vi "HEWH Standard ERD List.vi"(8 "Error In":errorcluster, 11 "Disable ERD (Main)":bool) -> (0 "Error Out":errorcluster, 2 "Header":string[](array[string]), 3 "Read ERD List":T1[](array[typedef]) {"ERD Number" format="%.0x"})   [LabVIEW 2016]
uses:
  type defs/ERD Read Data In.ctl
  type defs/Data Type.ctl
  library/GEA2_Toolkit.lvlib
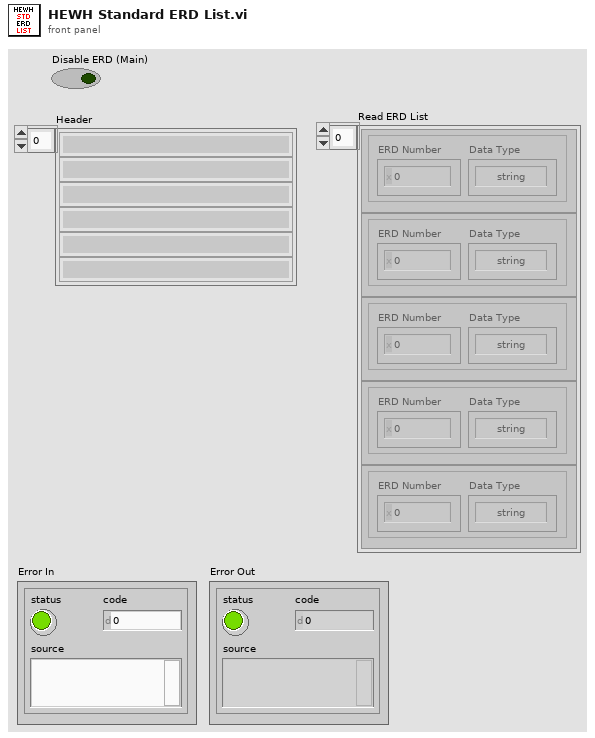
[diagram p1: front panel]
types:
  T1 = typedef "GEA2_Toolkit.lvlib/ERD Read Data In.ctl" = cluster{"ERD Number":u16, "Data Type":T2}
  T2 = typedef "GEA2_Toolkit.lvlib/Data Type.ctl" = enum16{"string", "boolean", "uint8_t", "uint16_t", "uint32_t", "uint64_t"}
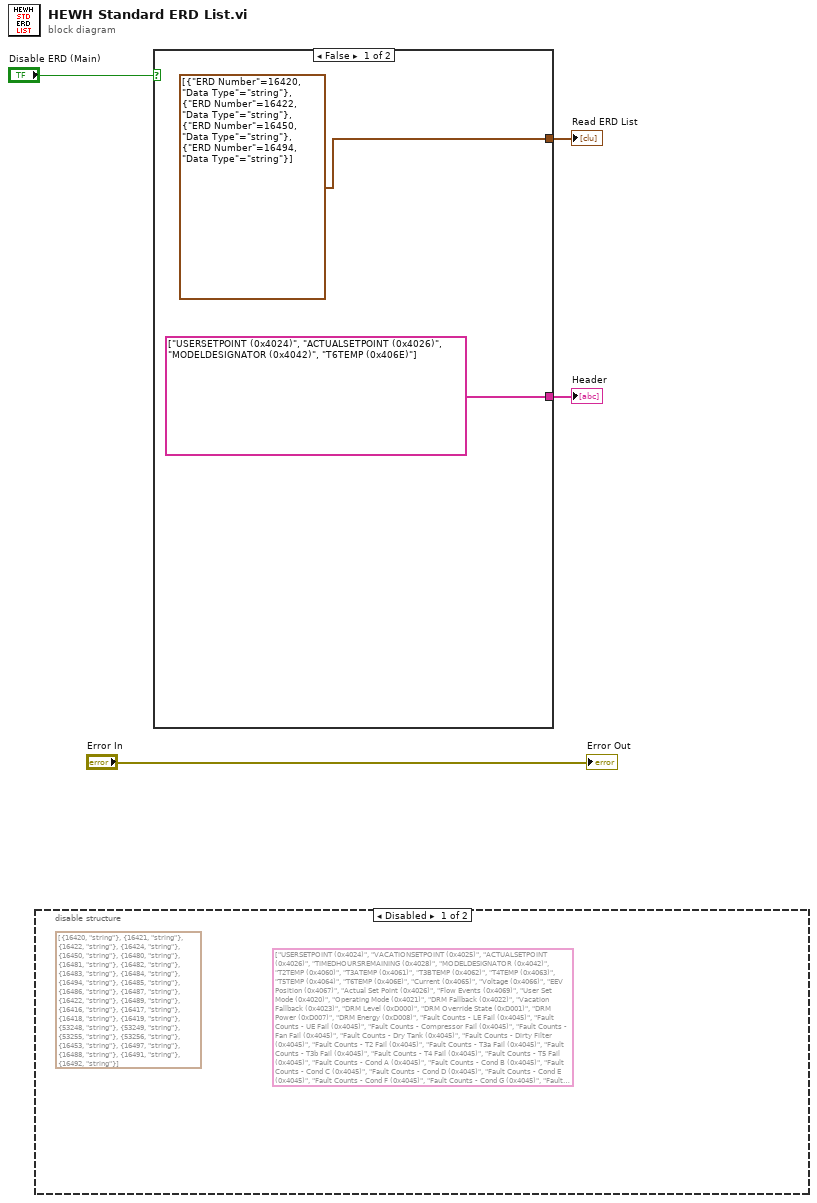
[diagram p0: block diagram]
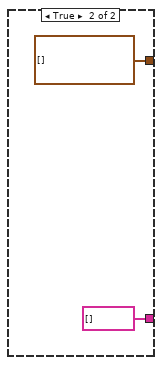
[diagram p3: hidden frame]
diagram:
  n1 = disable-structure shown="Disabled" {
    frame Disabled {
      (unwired) string[] ["USERSETPOINT (0x4024)", "VACATIONSETPOINT (0x4025)", "ACTUALSETPOINT (0x4026)", "TIMEDHOURSREMAINING (0x4028)", "MODELDESIGNATOR (0x4042)", "T2TEMP (0x4060)", "T3ATEMP (0x4061)", "T3BTEMP (0x4062)", "T4TEMP (0x4063)", "T5TEMP (0x4064)", "T6TEMP (0x406E)", "Current (0x4065)", "Voltage (0x4066)", "EEV Position (0x4067)", "Actual Set Point (0x4026)", "Flow Events (0x4069)", "User Set Mode (0x4020)", "Operating Mode (0x4021)", "DRM Fallback (0x4022)", "Vacation Fallback (0x4023)", "DRM Level (0xD000)", "DRM Override State (0xD001)", "DRM Power (0xD007)", "DRM Energy (0xD008)", "Fault Counts - LE Fail (0x4045)", "Fault Counts - UE Fail (0x4045)", "Fault Counts - Compressor Fail (0x4045)", "Fault Counts - Fan Fail (0x4045)", "Fault Counts - Dry Tank (0x4045)", "Fault Counts - Dirty Filter (0x4045)", "Fault Counts - T2 Fail (0x4045)", "Fault Counts - T3a Fail (0x4045)", "Fault Counts - T3b Fail (0x4045)", "Fault Counts - T4 Fail (0x4045)", "Fault Counts - T5 Fail (0x4045)", "Fault Counts - Cond A (0x4045)", "Fault Counts - Cond B (0x4045)", "Fault Counts - Cond C (0x4045)", "Fault Counts - Cond D (0x4045)", "Fault Counts - Cond E (0x4045)", "Fault Counts - Cond F (0x4045)", "Fault Counts - Cond G (0x4045)", "Fault Counts - Cond H (0x4045)", "Fault Counts - Cond I (0x4045)", "Fault Counts - Cond J (0x4045)", "Fault Counts - Cond L (0x4045)", "Condensate Drain Pan Voltage (0x4071)", "Relay States - DLB (0x4068)", "Relay States - Compressor (0x4068)", "Relay States - Upper Element (0x4068)", "Relay States - Lower Element (0x4068)", "Relay States - Fan (0x4068)", "Compressor Min On/Off Time (0x406B)", "SS Run State (0x406C)"]
      (unwired) T1[] [{"ERD Number"=16420, "Data Type"=enum."string"}, {"ERD Number"=16421, "Data Type"=enum."string"}, {"ERD Number"=16422, "Data Type"=enum."string"}, {"ERD Number"=16424, "Data Type"=enum."string"}, {"ERD Number"=16450, "Data Type"=enum."string"}, {"ERD Number"=16480, "Data Type"=enum."string"}, {"ERD Number"=16481, "Data Type"=enum."string"}, {"ERD Number"=16482, "Data Type"=enum."string"}, {"ERD Number"=16483, "Data Type"=enum."string"}, {"ERD Number"=16484, "Data Type"=enum."string"}, {"ERD Number"=16494, "Data Type"=enum."string"}, {"ERD Number"=16485, "Data Type"=enum."string"}, {"ERD Number"=16486, "Data Type"=enum."string"}, {"ERD Number"=16487, "Data Type"=enum."string"}, {"ERD Number"=16422, "Data Type"=enum."string"}, {"ERD Number"=16489, "Data Type"=enum."string"}, {"ERD Number"=16416, "Data Type"=enum."string"}, {"ERD Number"=16417, "Data Type"=enum."string"}, {"ERD Number"=16418, "Data Type"=enum."string"}, {"ERD Number"=16419, "Data Type"=enum."string"}, {"ERD Number"=53248, "Data Type"=enum."string"}, {"ERD Number"=53249, "Data Type"=enum."string"}, {"ERD Number"=53255, "Data Type"=enum."string"}, {"ERD Number"=53256, "Data Type"=enum."string"}, {"ERD Number"=16453, "Data Type"=enum."string"}, {"ERD Number"=16497, "Data Type"=enum."string"}, {"ERD Number"=16488, "Data Type"=enum."string"}, {"ERD Number"=16491, "Data Type"=enum."string"}, {"ERD Number"=16492, "Data Type"=enum."string"}] ("Read ERD List")
    }
    frame Enabled {
    }
  }
  n2 = case shown="False" "Disable ERD (Main)" {
    tunnel: [string[] ["USERSETPOINT (0x4024)", "ACTUALSETPOINT (0x4026)", "MODELDESIGNATOR (0x4042)", "T6TEMP (0x406E)"] string[] []] -> w4
    tunnel: [T1[] [{"ERD Number"=16420, "Data Type"=enum."string"}, {"ERD Number"=16422, "Data Type"=enum."string"}, {"ERD Number"=16450, "Data Type"=enum."string"}, {"ERD Number"=16494, "Data Type"=enum."string"}] ("Read ERD List") T1[] [] ("Read ERD List")] -> w3
    frame False {
    }
    frame True {
    }
  }
  "Header" <- w4
  "Read ERD List" <- w3
  "Error Out" <- "Error In"
